vi "Open.vi"(8 "error in (no error)":errorcluster) -> (0 "error out":errorcluster, 3 "VISA resource name out":refnum<visa-resource-name>)   [LabVIEW 2019]
uses:
  <vilib>/Instr/_visa.llb/VISA Configure Serial Port (Instr).vi
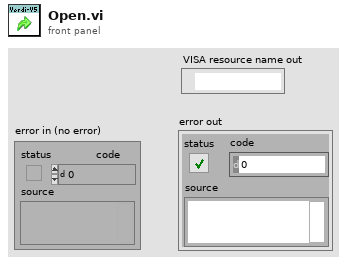
[diagram p1: front panel]
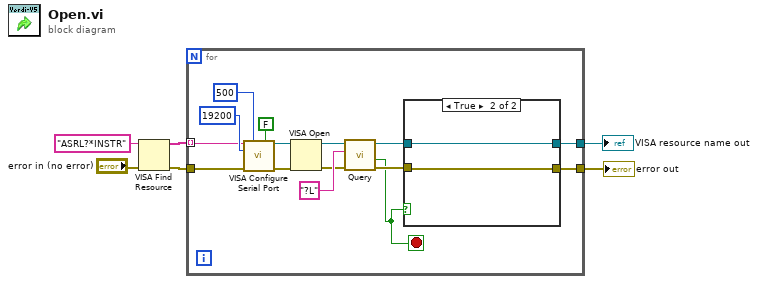
[diagram p0: block diagram]
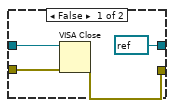
[diagram p2: hidden frame]
diagram:
  n1 = VISA Find Resource(8:"error in (no error)", 11:"ASRL?*INSTR" ("expression (\"?*\")")) -> (0:w2:errorcluster, 3:w3:string[])  [unwired: 1 in, 1 out]
  n2 = for {
    tunnel: w3 -> [w17] mode=indexing
    tunnel: [w13] -> w4
    tunnel: [w12] -> w5
    tunnel: w2 -> [w10]
    stop <- w7 stop-if-true
    n3 = call-poly "VISA Configure Serial Port"("VISA resource name"=w17, "timeout (10sec)"=u32 500, "Enable Termination\nChar (T)"=FALSE ("Enable Termination\nChar (T)"), "baud rate (9600)"=u32 19200, "error in (no error)"=w10) -> ("VISA resource name out"=w21:refnum<visa-resource-name>, "error out"=w16:errorcluster)  [unwired: 9 in]
    n4 = VISA Open(error in (no error)=w16, VISA resource name=w21) -> (VISA resource name=w9:refnum<visa-resource-name>, error out=w8:errorcluster)  [unwired: 3 in]
    n5 = call "Query.vi"("error in (no error)"=w8, "Command"="?L", "VISA resource name"=w9) -> ("error out"=w11:errorcluster, "Resp?"=w7:bool, "VISA resource name out"=w14:refnum<visa-resource-name>)  [unwired: 5 in, 1 out]
    n6 = case shown="True" w7 {
      tunnel: w14 -> [w24 w27]
      tunnel: [refnum<visa-resource-name> refnum ("VISA resource name out") w27] -> w13
      tunnel: w11 -> [w23 w26]
      tunnel: [w22 w26] -> w12
      frame False {
        n7 = VISA Close(VISA resource name=w24, error in (no error)=w23) -> (error out=w22:errorcluster)
      }
      frame True {
      }
    }
  }
  "VISA resource name out" <- w4
  "error out" <- w5
